vi "Properties to String.vi"(1 "Properties":T1[](array[typedef])) -> (0 "String":string)   [LabVIEW 2015, in "JFrog CLI.lvclass"]
uses:
  JFrog CLI.lvclass
  Typedef/Property.ctl
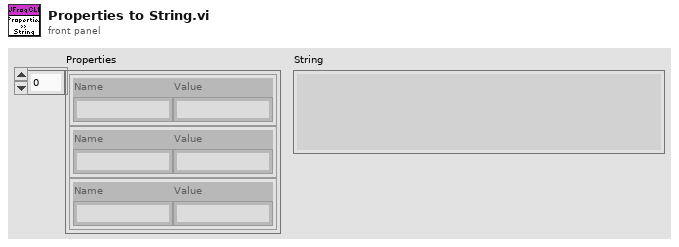
[diagram p1: front panel]
types:
  T1 = typedef "JFrog CLI.lvclass/Property.ctl" = cluster{"Name":string, "Value":string}
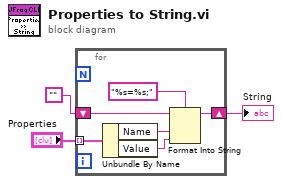
[diagram p0: block diagram]
diagram:
  n1 = for {
    tunnel: "Properties" -> [w9] mode=indexing
    shift-right: [w4] -> w1
    shift-left: "" -> [w5]
    n2 = Unbundle By Name(w9) -> ("Name"=w8:string, "Value"=w7:string)
    n3 = Format Into String(format string="%s=%s;", initial string=w5, w8, w7) -> (resulting string=w4:string)  [unwired: 1 in, 1 out]
  }
  "String" <- w1
